vi "GetDataFromString.vi"(0 "strArrayIn":string[](array[string])) -> (1 "strArrayBuf":string[](array[string]), 2 "mu32ArrayOut":u32[](array[numeric]))   [LabVIEW 2011]
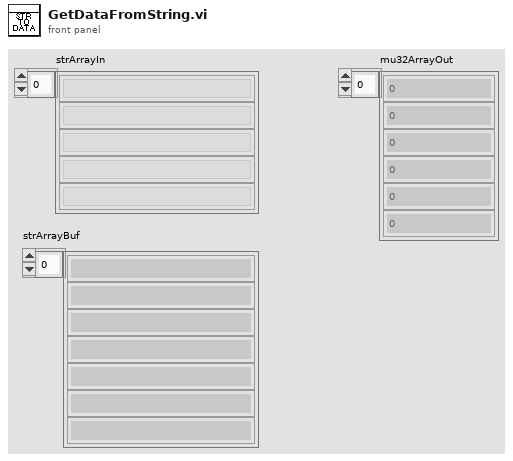
[diagram p1: front panel]
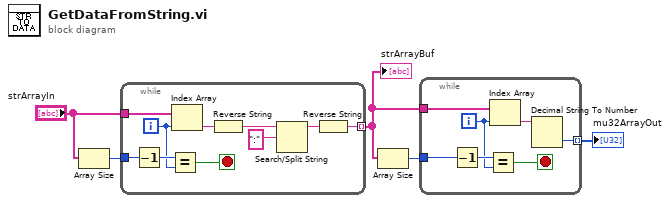
[diagram p0: block diagram]
diagram:
  n1 = Array Size(array="strArrayIn") -> (size(s)=w5:i32)
  n2 = while {
    tunnel: w5 -> [w14]
    tunnel: "strArrayIn" -> [w12]
    tunnel: [w6] -> w1 mode=indexing
    i -> [w7]
    stop <- w15 stop-if-true
    n3 = Decrement(x=w14) -> (x-1=w13:i32)
    n4 = Equal?(x=w13, y=w7) -> (x = y?=w15:bool)
    n5 = Index Array(array=w12, index=w7) -> (element=w11:string)
    n6 = Reverse String(1:w11) -> (0:w10:string)
    n7 = Search/Split String(string=w10, search string/char (-)=":" ("搜索字符串/字符(-)")) -> (substring before match=w8:string)  [unwired: 1 in, 2 out]
    n8 = Reverse String(1:w8) -> (0:w6:string)
  }
  "strArrayBuf" <- w1
  n9 = Array Size(array=w1) -> (size(s)=w3:i32)
  n10 = while {
    tunnel: w3 -> [w22]
    tunnel: w1 -> [w18]
    tunnel: [w16] -> w2 mode=indexing
    i -> [w19]
    stop <- w20 stop-if-true
    n11 = Decrement(x=w22) -> (x-1=w21:i32)
    n12 = Equal?(x=w21, y=w19) -> (x = y?=w20:bool)
    n13 = Index Array(array=w18, index=w19) -> (element=w17:string)
    n14 = Decimal String To Number(string=w17) -> (number=w16:i32)  [unwired: 2 in, 1 out]
  }
  "mu32ArrayOut" <- w2
